vi "Sequence.Parameterize.vi"(8 "error in (no error)":errorcluster, 10 "Station.ID":string, 11 "Sequence":refnum<k24>) -> (0 "error out":errorcluster, 3 "Sequence":refnum<k24>)   [LabVIEW 2015, in "Single Station Execution.lvlib"]
uses:
  Single Station Execution.lvlib
  NationalInstruments.VeriStand.RealTimeSequenceDefinitionApi
  NationalInstruments.VeriStand.DataTypes
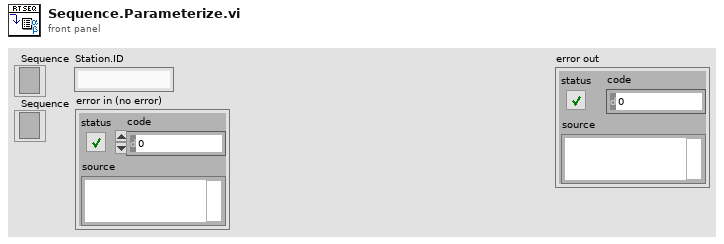
[diagram p1: front panel]
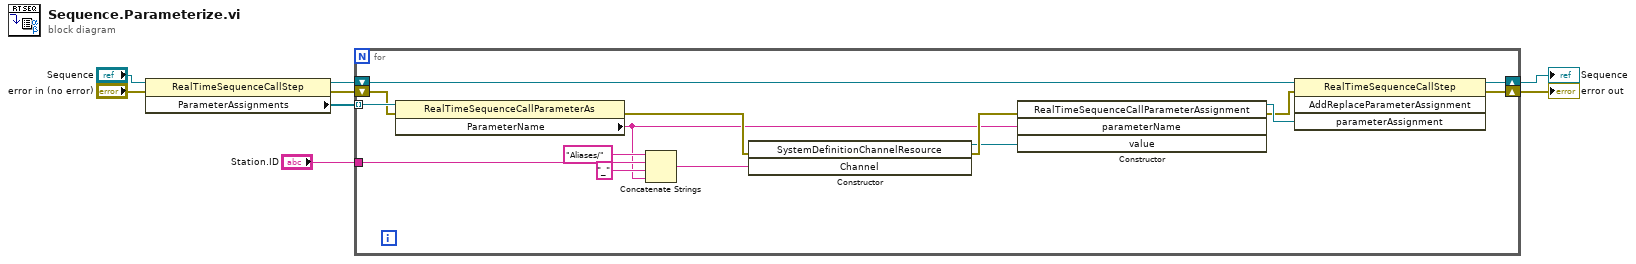
[diagram p0: block diagram]
diagram:
  n1 = property class="RealTimeSequenceCallStep"(reference="Sequence", error in="error in (no error)") -> (reference out=w5:refnum<k24>, error out=w3:errorcluster, "ParameterAssignments"=w7:refnum<k24>[])
  n2 = for {
    tunnel: w7 -> [w23] mode=indexing
    tunnel: "Station.ID" -> [w21]
    shift-right: [w11] -> w4
    shift-left: w5 -> [w19]
    shift-right: [w10] -> w2
    shift-left: w3 -> [w9]
    n3 = property class="RealTimeSequenceCallParameterAs"(reference=w23, error in=w9) -> (error out=w15:errorcluster, "ParameterName"=w12:string)  [unwired: 1 out]
    n4 = Concatenate Strings("Aliases/" ("string"), w21, "_" ("string"), w12) -> (w16:string)
    n5 = constructor class="SystemDefinitionChannelResource"(error in=w15, "Channel"=w16) -> (reference out=w13:refnum<k24>, error out=w14:errorcluster)  [unwired: 2 in, 2 out]
    n6 = constructor class="RealTimeSequenceCallParameterAs"(error in=w14, "parameterName"=w12, "value"=w13) -> (reference out=w18:refnum<k24>, error out=w17:errorcluster)  [unwired: 2 in, 3 out]
    n7 = invoke class="RealTimeSequenceCallStep" method="AddReplaceParameterAssignment"(reference=w19, error in=w17, "parameterAssignment"=w18) -> (reference out=w11:refnum<k24>, error out=w10:errorcluster)  [unwired: 1 in, 2 out]
  }
  "Sequence" <- w4
  "error out" <- w2
